vi "Charm Variables.vi"() -> (1 "Charm Width":i32=646, 2 "Charm Peek Width":u32=15)   [LabVIEW 2012, in "Win8uiFramework.lvlib" / "MainController.lvclass"]
uses:
  MainController.lvclass
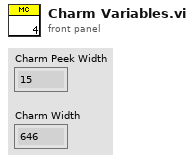
[diagram p1: front panel]
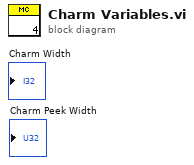
[diagram p0: block diagram]
diagram:
